vi "DBM Pannel Size.vi"(4 "TBCALSTD_temp":refnum<vi>, 5 "새로고침 2":refnum<vi>, 6 "tbl 참조 배열":refnum<vi>[](array[refnum]), 7 "모델등록요청LIST 2":refnum<vi>, 8 "에러 입력":errorcluster caption="에러 입력(에러 없음)", 9 "참조 배열":refnum<vi>[](array[refnum]), 10 "TabCtl 참조 번호":refnum<vi>, 11 "Slide 입력":refnum<vi>) -> (0 "에러 출력":errorcluster)   [LabVIEW 2020]
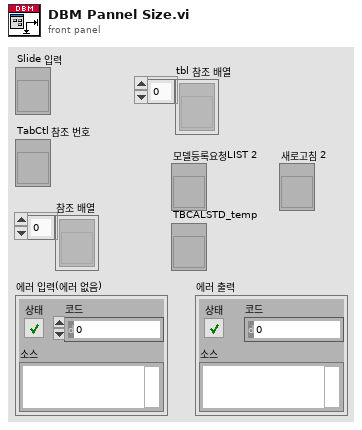
[diagram p1: front panel]
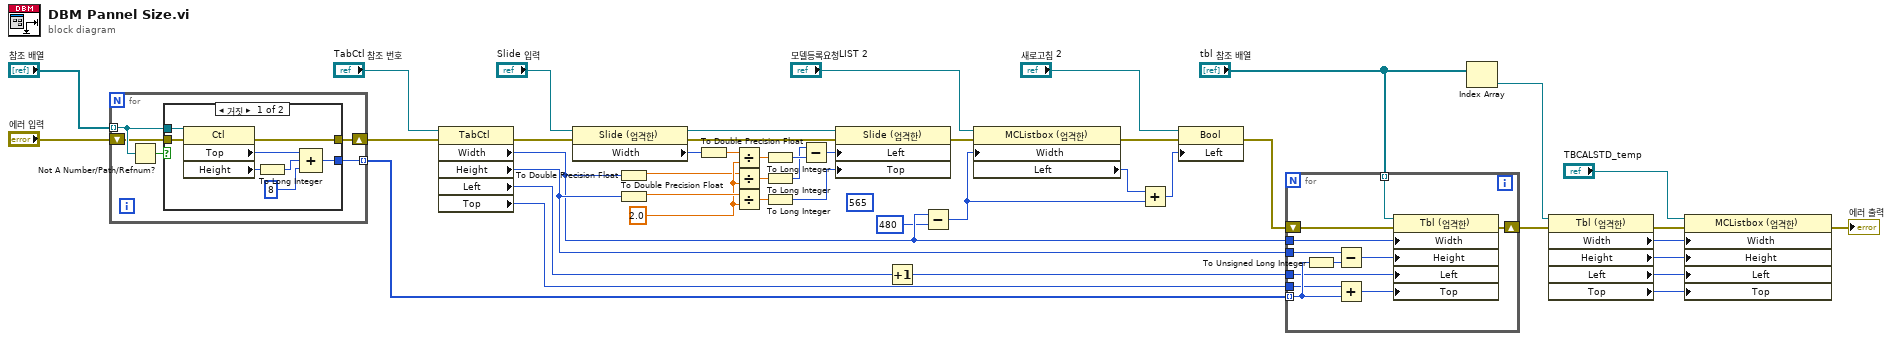
[diagram p0: block diagram]
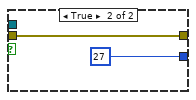
[diagram p2: hidden frame]
diagram:
  (unwired) u32 565 ("y")
  w37 = 2.0 ("y")
  n1 = for {
    tunnel: "참조 배열" -> [w50] mode=indexing
    tunnel: [w48] -> w21 mode=indexing
    shift-right: [w46] -> w22
    shift-left: "에러 입력" -> [w47]
    n2 = Not A Number/Path/Refnum?(number/path/refnum=w50) -> (NaN/Path/Refnum?=w49:bool)
    n3 = case shown="거짓" w49 {
      tunnel: w50 -> [w58 _]
      tunnel: [w53 27] -> w48
      tunnel: w47 -> [w52 w59]
      tunnel: [w51 w59] -> w46
      frame False {
        n4 = property class="Ctl"(reference=w58, error in=w52) -> (error out=w51:errorcluster, "Top"=w54:i32, "Height"=w55:u32)  [unwired: 1 out]
        n5 = To Long Integer(number=w55) -> (32bit integer=w56:i32)
        n6 = Compound Arithmetic op=ADD(w54, w56, 8 ("y")) -> (w53:i32)
      }
      frame True {
      }
    }
  }
  n7 = property on="프로퍼티 노드" class="TabCtl"(reference="TabCtl 참조 번호", error in=w22) -> (error out=w43:errorcluster, "Width"=w18:u32, "Height"=w31:u32, "Left"=w29:i32, "Top"=w30:i32)  [unwired: 1 out]
  n8 = property on="프로퍼티 노드" class="Slide (엄격한)"(reference="Slide 입력", error in=w43) -> (reference out=w26:refnum<vi>, error out=w44:errorcluster, "Width"=w45:u32)
  n9 = To Double Precision Float(number=w18) -> (double precision float=w35:dbl)
  n10 = To Double Precision Float(number=w31) -> (double precision float=w41:dbl)
  n11 = To Double Precision Float(number=w45) -> (double precision float=w36:dbl)
  n12 = Divide(x=w36, y=w37) -> (x/y=w39:dbl)
  n13 = Divide(x=w35, y=w37) -> (x/y=w33:dbl)
  n14 = Divide(x=w41, y=w37) -> (x/y=w32:dbl)
  n15 = To Long Integer(number=w39) -> (32bit integer=w40:i32)
  n16 = To Long Integer(number=w33) -> (32bit integer=w34:i32)
  n17 = To Long Integer(number=w32) -> (32bit integer=w42:i32)
  n18 = Subtract(x=w34, y=w40) -> (x-y=w38:i32)
  n19 = property on="프로퍼티 노드" class="Slide (엄격한)"(reference=w26, error in=w44, "Left"=w38, "Top"=w42) -> (error out=w19:errorcluster)  [unwired: 1 out]
  n20 = Increment(x=w29) -> (x+1=w25:i32)
  n21 = Subtract(x=w18, y=u32 480) -> (x-y=w11:u32)
  n22 = property on="프로퍼티 노드" class="MCListbox (엄격한)"(reference="모델등록요청LIST 2", error in=w19, "Width"=w11) -> (error out=w15:errorcluster, "Left"=w12:i32)  [unwired: 1 out]
  n23 = Add(x=w12, y=w11) -> (x+y=w13:u32)
  n24 = property class="Bool"(reference="새로고침 2", error in=w15, "Left"=w13) -> (error out=w14:errorcluster)  [unwired: 1 out]
  n25 = for {
    tunnel: w21 -> [w68] mode=indexing
    shift-right: [w71] -> w8
    shift-left: w14 -> [w70]
    tunnel: "tbl 참조 배열" -> [w65] mode=indexing
    tunnel: w18 -> [w64]
    tunnel: w31 -> [w63]
    tunnel: w25 -> [w62]
    tunnel: w30 -> [w61]
    n26 = To Unsigned Long Integer(number=w68) -> (unsigned 32bit integer=w67:u32)
    n27 = Subtract(x=w63, y=w67) -> (x-y=w66:u32)
    n28 = Add(x=w61, y=w68) -> (x+y=w69:i32)
    n29 = property class="Tbl (엄격한)"(reference=w65, error in=w70, "Width"=w64, "Height"=w66, "Left"=w62, "Top"=w69) -> (error out=w71:errorcluster)  [unwired: 1 out]
  }
  n30 = Index Array(array="tbl 참조 배열") -> (element=w9:refnum<vi>)  [unwired: 1 in]
  n31 = property class="Tbl (엄격한)"(reference=w9, error in=w8) -> (error out=w7:errorcluster, "Width"=w4:u32, "Height"=w3:u32, "Left"=w2:i32, "Top"=w1:i32)  [unwired: 1 out]
  n32 = property class="MCListbox (엄격한)"(reference="TBCALSTD_temp", error in=w7, "Width"=w4, "Height"=w3, "Left"=w2, "Top"=w1) -> (error out=→"에러 출력":errorcluster)  [unwired: 1 out]
